vi "Read UI Refnum.vi"(8 "error in (no error)":errorcluster, 11 "Project in":refnum<class "Project.lvclass">) -> (0 "error out":errorcluster, 2 "VI Refnum":refnum<vi>, 3 "Project out":refnum<class "Project.lvclass">)   [LabVIEW 2015, in "Project.lvclass"]
uses:
  Project.lvclass
  Project Configure UI.vi
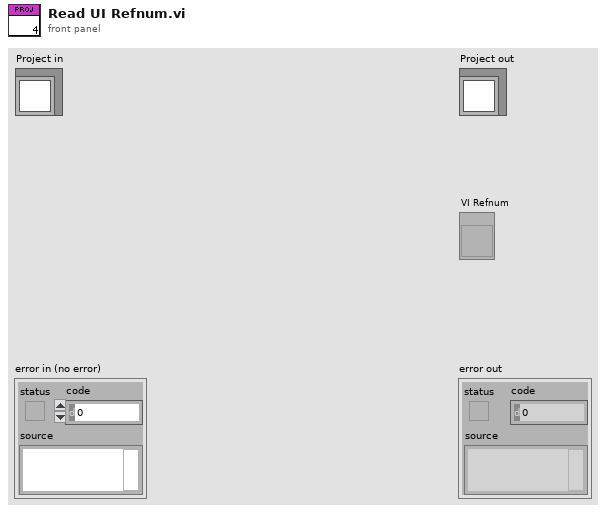
[diagram p1: front panel]
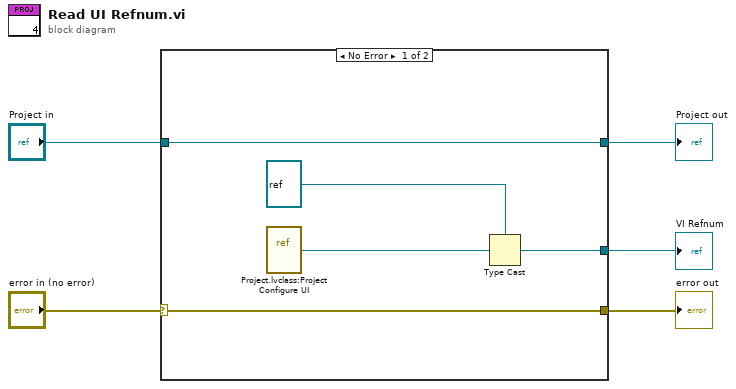
[diagram p0: block diagram]
diagram:
  n1 = case shown="No Error" "error in (no error)" {
    selector: "error in (no error)" -> [w10 w11]
    tunnel: [w10 w11] -> w4
    tunnel: "Project in" -> [w7 w12]
    tunnel: [w7 w12] -> w2
    tunnel: [w6 _] -> w1
    frame No Error {
      n2 = vi-ref "Project.lvclass:Project Configure UI.vi"() -> (w8:refnum<vi>)
      n3 = Type Cast(type=refnum<vi> refnum ("vi reference"), x=w8) -> (*(type *) &x=w6:refnum<vi>)
    }
    frame Error {
    }
  }
  "error out" <- w4
  "Project out" <- w2
  "VI Refnum" <- w1
